vi "After Launch Init.vi"(8 "error in (no error)":errorcluster, 11 "CS++Fgen in":refnum<class "CS++Fgen.lvclass">) -> (0 "error out":errorcluster, 3 "CS++Fgen out":refnum<class "CS++Fgen.lvclass">)   [LabVIEW 2013, in "CS++Fgen.lvlib" / "CS++Fgen.lvclass"]
doc: "Use <b>Pre Launch init.vi</b> method for sanity checks that are supposed to prevent the actor from launching if they fail. Use <B>this</B> method instead to initialize this actor when it has been activated. A corresponding high priority message will become dispatched before the <B>Actor Core.vi</b> is called.\n\n<b>Derived classed should call the parent methode first</b> and their own initialization code after.\n\nRefer also to the ongoing discussion at https://decibel.ni.com/content/message/57394#57394."
uses:
  CS++Fgen.lvclass
  CSPP_Core/Classes/CS++ProcessVariables/ProcessVariable/PV.lvclass
  CS++Fgen.lvclass/CS++Fgen.ctl
  CSPP_Core/Classes/CS++ProcessVariables/PVConnection/PVConnection.lvclass
  CSPP_Core/Classes/CS++ProcessVariables/ProcessVariable/PV.lvclass/PV.ctl
  CSPP_Core/Actors/CS++DeviceActor/CS++DeviceActor.lvclass
  CSPP_Core/Classes/CS++ProcessVariables/ProcessVariable/Write Data.vi
  CSPP_Core/Classes/CS++ProcessVariables/ProcessVariable/Write Error.vi
  CSPP_Core/Classes/CS++ProcessVariables/ProcessVariable/Write Quality.vi
  CSPP_Core/Classes/CS++ProcessVariables/ProcessVariable/Write status.vi
  CSPP_Core/Classes/CS++ProcessVariables/ProcessVariable/Write Timestamp.vi
  <vilib>/ActorFramework/Actor/Actor.lvclass
  <vilib>/ActorFramework/Message/Message.lvclass
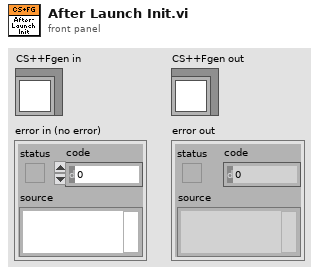
[diagram p1: front panel]
types:
  T1 = cluster{"Write Access":enum8{"Allowed", "Required", "None"}, "Read Access":enum8{"Allowed", "Required", "None"}}
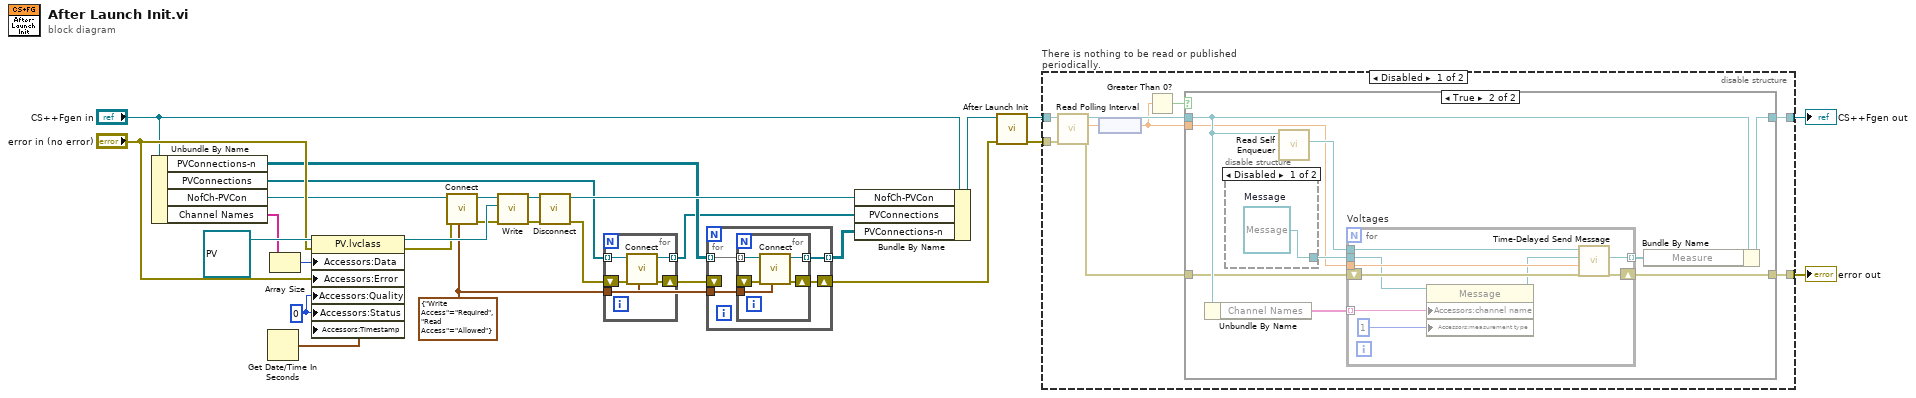
[diagram p0: block diagram]
diagram:
  w6 = T1 {"Write Access"=enum."Required", "Read Access"=enum."Allowed"} ("Access")
  w24 = 0 ("Quality")
  n1 = Unbundle By Name("CS++Fgen in") -> ("PVConnections-n"=w8:refnum<class "PVConnection.lvclass">[][], "PVConnections"=w7:refnum<class "PVConnection.lvclass">[], "NofCh-PVCon"=w15:refnum<class "PVConnection.lvclass">, "Channel Names"=w21:string[])
  n2 = Get Date/Time In Seconds() -> (seconds since 1Jan1904=w25:timestamp)
  n3 = Array Size(array=w21) -> (size(s)=w23:i32)
  n4 = property class="PV.lvclass"(reference=refnum<class "PV.lvclass"> refnum ("CS++ProcessVariables.lvlib:PV.lvclass"), error in="error in (no error)", "Accessors:Data"=w23, "Accessors:Error"="error in (no error)", "Accessors:Quality"=w24, "Accessors:Status"=w24, "Accessors:Timestamp"=w25) -> (reference out=w26:refnum<class "PV.lvclass">, error out=w12:errorcluster)
  n5 = call-dynamic "Connect.vi"("Access (R/W allowed)"=w6, "error in (no error)"=w12, "PVConnection in"=w15) -> ("error out"=w13:errorcluster, "PVConnection out"=w14:refnum<class "PVConnection.lvclass">)  [unwired: 7 in]
  n6 = call-dynamic "Write.vi"("error in (no error)"=w13, "PV"=w26, "PVConnection in"=w14) -> ("error out"=w28:errorcluster, "PVConnection out"=w27:refnum<class "PVConnection.lvclass">)  [unwired: 7 in]
  n7 = call-dynamic "Disconnect.vi"("error in (no error)"=w28, "PVConnection in"=w27) -> ("error out"=w2:errorcluster, "PVConnection out"=w9:refnum<class "PVConnection.lvclass">)  [unwired: 8 in]
  n8 = for {
    tunnel: w7 -> [w33] mode=indexing
    tunnel: [w32] -> w4 mode=indexing
    tunnel: w6 -> [w31]
    shift-right: [w30] -> w5
    shift-left: w2 -> [w29]
    n9 = call-dynamic "Connect.vi"("Access (R/W allowed)"=w31, "error in (no error)"=w29, "PVConnection in"=w33) -> ("error out"=w30:errorcluster, "PVConnection out"=w32:refnum<class "PVConnection.lvclass">)  [unwired: 7 in]
  }
  n10 = for {
    tunnel: w6 -> [w37]
    tunnel: w8 -> [w36] mode=indexing
    tunnel: [w35] -> w3 mode=indexing
    shift-right: [w34] -> w1
    shift-left: w5 -> [_]
    n11 = for {
      tunnel: w36 -> [w42] mode=indexing
      tunnel: [w41] -> w35 mode=indexing
      tunnel: w37 -> [w40]
      shift-right: [w39] -> w34
      shift-left: _ -> [w38]
      n12 = call-dynamic "Connect.vi"("Access (R/W allowed)"=w40, "error in (no error)"=w38, "PVConnection in"=w42) -> ("error out"=w39:errorcluster, "PVConnection out"=w41:refnum<class "PVConnection.lvclass">)  [unwired: 7 in]
    }
  }
  n13 = Bundle By Name(cluster="CS++Fgen in", "NofCh-PVCon"=w9, "PVConnections"=w4, "PVConnections-n"=w3) -> (w10:refnum<class "CS++Fgen.lvclass">)
  n14 = call-parent "After Launch Init.vi"("error in (no error)"=w1, "CS++DeviceActor in"=w10) -> ("error out"=w18:errorcluster, "CS++DeviceActor out"=w19:refnum<class "CS++Fgen.lvclass">)  [unwired: 8 in]
  n15 = disable-structure "There is nothing to be read or published periodically." shown="Disabled" {
    disable-tunnel: w19 -> [w46 w74]
    disable-tunnel: w18 -> [w45 w73]
    disable-tunnel: [w44 w74] -> w17
    disable-tunnel: [w43 w73] -> w16
    frame Disabled {
      n16 = call "Read Polling Interval.vi"("error in (no error)"=w45, "CS++DeviceActor in"=w46) -> ("error out"=w50:errorcluster, "Polling Interval"=w49:dbl[unit], "CS++DeviceActor out"=w51:refnum<class "CS++Fgen.lvclass">)  [unwired: 7 in]
      n17 = node(w49) -> (w48:dbl)
      n18 = Greater Than 0?(x=w48) -> (x > 0?=w47:bool)
      n19 = case shown="True" w47 {
        tunnel: [w53 w62] -> w44
        tunnel: [w52 w54] -> w43
        tunnel: w51 -> [w53 w61]
        tunnel: w50 -> [w52 w58]
        tunnel: w48 -> [_ w57]
        frame False {
        }
        frame True {
          n20 = Unbundle By Name(w61) -> ("Channel Names"=w56:string[])
          n21 = disable-structure shown="Disabled" {
            disable-tunnel: [w63 _] -> w60
            frame Disabled {
              w63 = refnum<class "Message.lvclass"> refnum  # Message
            }
            frame Enabled {
            }
          }
          n22 = call <vilib>:"Read Self Enqueuer.vi"("Actor"=w61) -> ("Self Enqueuer"=w59:refnum<class "Message Enqueuer.lvclass">)  [unwired: 10 in]
          n23 = for "Voltages" {
            tunnel: w59 -> [w71]
            tunnel: w57 -> [w69]
            tunnel: [w68] -> w55 mode=indexing
            tunnel: w60 -> [w64]
            shift-right: [w72] -> w54
            shift-left: w58 -> [w70]
            tunnel: w56 -> [w67] mode=indexing
            n24 = property class="Message"(reference=w64, "Accessors:channel name"=w67, "Accessors:measurement type"=1 ("measurement type (voltage)")) -> (reference out=w65:refnum<class "Message.lvclass">)  [unwired: 1 in, 1 out]
            n25 = call <vilib>:"Time-Delayed Send Message.vi"("error in (no error)"=w70, "Milliseconds To Wait"=w69, "Message"=w65, "Message Enqueuer"=w71) -> ("error out"=w72:errorcluster, "Delivery Notifier"=w68:refnum<notifier>)  [unwired: 6 in]
          }
          n26 = Bundle By Name(cluster=w61, "Measure"=w55) -> (w62:refnum<class "CS++Fgen.lvclass">)
        }
      }
    }
    frame Enabled {
    }
  }
  "error out" <- w16
  "CS++Fgen out" <- w17
